vi "subvi1.vi"() -> (3 "VI Path":path)   [LabVIEW 2017]
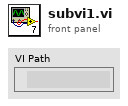
[diagram p1: front panel]
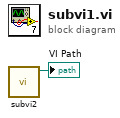
[diagram p0: block diagram]
diagram:
  n1 = call "subvi2.vi"() -> ("VI Path"=→"VI Path":path)  [unwired: 11 in]
